vi "AH2700_write_data.vi"   [LabVIEW 2016]
uses:
  Global/Global Variables/global.vi
  CryoTUM-V1.0/Instrument_Setup.vi
  Global/Global Variables/Data_Display_global.vi
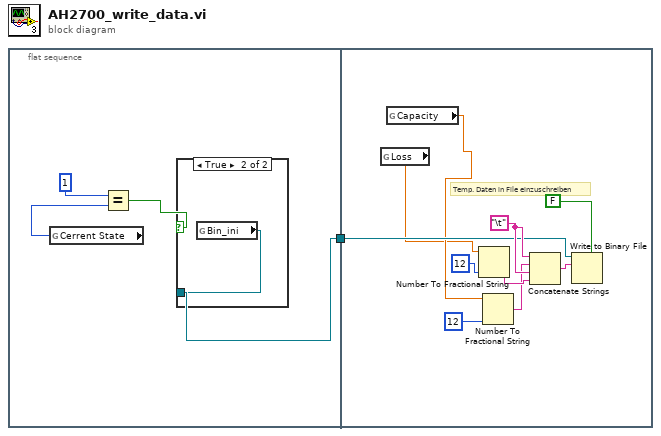
[diagram p0: block diagram]
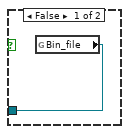
[diagram p2: hidden frame]
diagram:
  n1 = flat-sequence {
    tunnel: [w2] -> w1
    tunnel: w1 -> [w10]
    frame #0 {
      n2 = global read "global.vi" "Cerrent State"() -> (w4:i32)
      n3 = Equal?(x=1, y=w4) -> (x = y?=w3:bool)
      n4 = case shown="True" w3 {
        tunnel: [w6 w7] -> w2
        frame False {
          n5 = global read "Instrument_Setup.vi" "Bin_file"() -> (w6:refnum<file>)
        }
        frame True {
          n6 = global read "Instrument_Setup.vi" "Bin_ini"() -> (w7:refnum<file>)
        }
      }
    }
    frame #1 {
      w15 = "\t"
      # "Temp. Daten in File einzuschreiben"
      n7 = global read "Data_Display_global.vi" "Loss"() -> (w8:dbl)
      n8 = global read "Data_Display_global.vi" "Capacity"() -> (w9:dbl)
      n9 = Number To Fractional String(number=w8, precision (6)=i16 12) -> (F-format string=w16:string)  [unwired: 2 in]
      n10 = Number To Fractional String(number=w9, precision (6)=i16 12) -> (F-format string=w12:string)  [unwired: 2 in]
      n11 = Concatenate Strings(w15, w12, w15, w16) -> (w17:string)
      n12 = Write to Binary File ("Write File")(file (use dialog)=w10, data=w17, 5:FALSE ("prepend array or string size? (T)")) -> ()  [unwired: 3 in, 3 out]
    }
  }
